vi "tilt.vi"(8 "error in (no error)":errorcluster, 10 "angle":dbl[unit], 11 "GenericTrajectory in":refnum<class "TrajectoryDL091126GenericVoxel.lvclass">) -> (0 "error out":errorcluster, 3 "GenericTrajectory out":refnum<class "TrajectoryDL091126GenericVoxel.lvclass">)   [LabVIEW 2010, in "TrajectoryDL091126GenericVoxel.lvclass"]
uses:
  TrajectoryDL091126GenericVoxel.lvclass
  TrajectoryDL091126GenericVoxel.lvclass/TrajectoryDL091126GenericVoxel.ctl
  common/legacy/axes.ctl
  common/enumerations/x_y_z_enumeration.ctl
  common/enumerations/functional_global_action_enum.ctl
  <vilib>/express/express arith-compare/Formula/XNode/ExpressFormulaBlockNode.xnode
  <vilib>/Analysis/Matrix/Numeric/Conversions/Array To Matrix - RA2.vi
  <vilib>/Analysis/baseanly.llb/Real A x B.vi
  <vilib>/Analysis/Matrix/Numeric/Conversions/Matrix To Array - RM.vi
  common/classes/ErrorController/ErrorController/class_data.vi
  <vilib>/Analysis/Matrix/NI_Matrix.lvlib
  <vilib>/Analysis/NI_AALBase.lvlib
  common/classes/ErrorController/ErrorController/ErrorController.lvclass
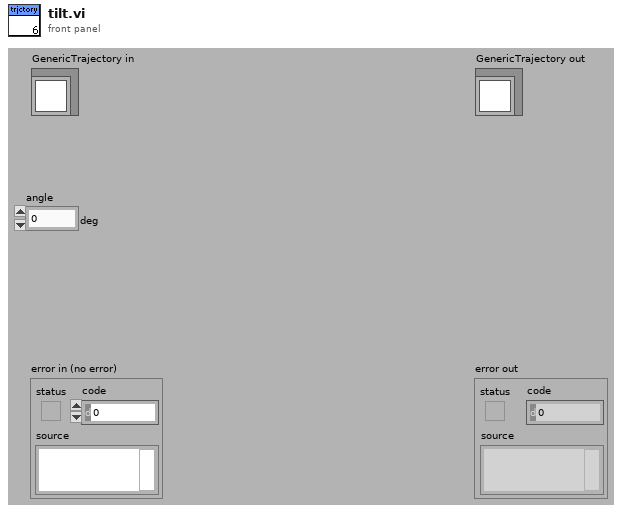
[diagram p1: front panel]
types:
  T1 = typedef "axes.ctl" = enum16{"x", "y", "z"}
  T2 = typedef "x_y_z_enumeration.ctl" = enum16{"x", "y", "z"}
  T3 = typedef "functional_global_action_enum.ctl" = enum16{"get", "set", "reset"}
  T4 = typedef "NI_Matrix.lvlib/RealMatrix.ctl" = dbl[][]
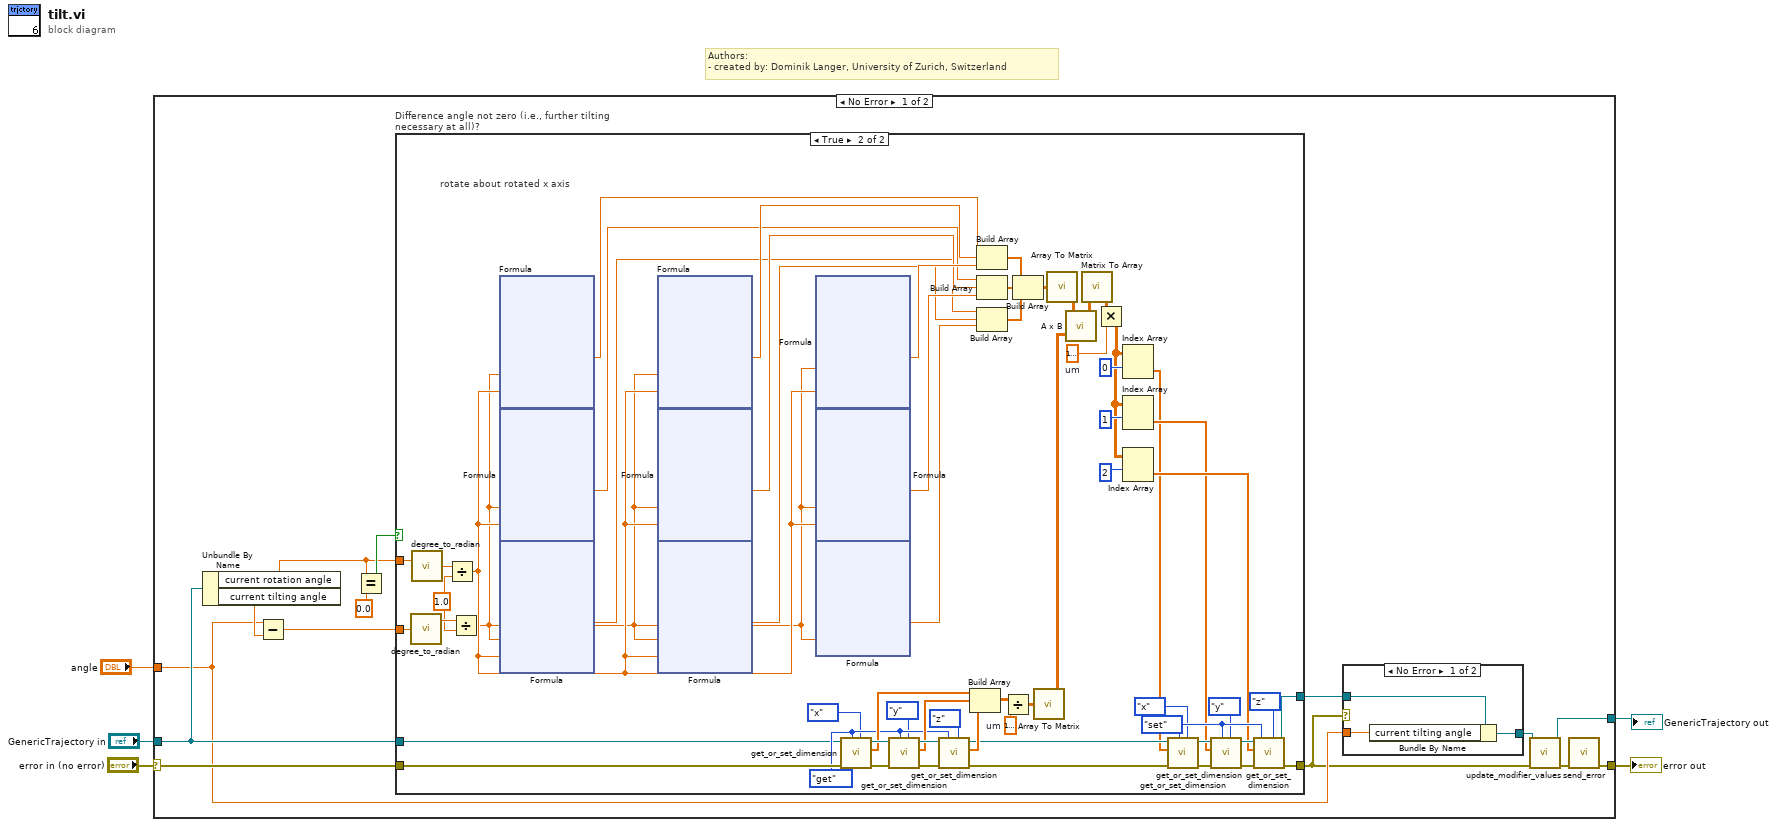
[diagram p0: block diagram]
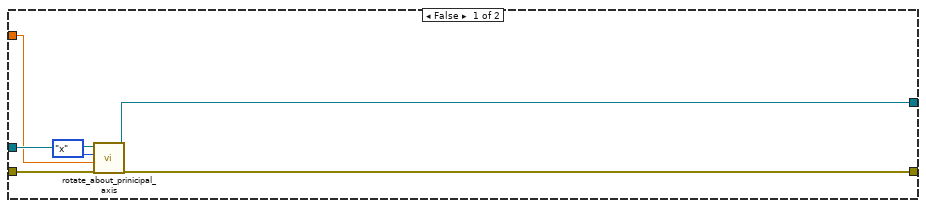
[diagram p3: hidden frame]
diagram:
  # "Authors: \n- created by: Dominik Langer, University of Zurich, Switzerland"
  n1 = case shown="No Error" "error in (no error)" {
    selector: "error in (no error)" -> [w15 w178]
    tunnel: [w6 w178] -> w4
    tunnel: [w8 w177] -> w2
    tunnel: "GenericTrajectory in" -> [w13 w177]
    tunnel: "angle" -> [w11 _]
    frame No Error {
      n2 = Unbundle By Name(w13) -> ("current rotation angle"=w14:dbl[unit], "current tilting angle"=w17:dbl[unit])
      n3 = Subtract(x=w11, y=w17) -> (x-y=w16:dbl[unit])
      n4 = Equal?(x=w14, y=dbl[unit] 0.0) -> (x = y?=w18:bool)
      n5 = case "Difference angle not zero (i.e., further tilting necessary at all)?" shown="True" w18 {
        tunnel: w16 -> [w24 w67]
        tunnel: w15 -> [w28 w60]
        tunnel: w13 -> [w26 w52]
        tunnel: w14 -> [_ w69]
        tunnel: [w25 w43] -> w12
        tunnel: [w27 w46] -> w10
        frame False {
          n6 = call-dynamic "rotate_about_prinicipal_axis.vi"("error in (no error)"=w28, "angle"=w24, "axis"=axes."x", "GenericTrajectory in"=w26) -> ("error out"=w27:errorcluster, "GenericTrajectory out"=w25:refnum<class "TrajectoryDL091126GenericVoxel.lvclass">)  [unwired: 6 out]
        }
        frame True {
          w49 = functional_global_action_enum."set" ("action")
          w54 = functional_global_action_enum."get" ("action")
          w66 = dbl[unit] 1.0 ("y")
          w38 = dbl[unit] 1e-06  # um
          w71 = dbl[unit] 1e-06  # um
          # "rotate about rotated x axis"
          n7 = call "degree_to_radian.vi"("angle in"=w67) -> ()  [unwired: 1 out]
          n8 = call "degree_to_radian.vi"("angle in"=w69) -> ("angle out"=w68:dbl[unit])
          n9 = Divide(x=w68, y=w66) -> (x/y=w70:dbl)
          n10 = Divide(x=w67, y=w66) -> (x/y=w65:dbl)
          n11 = xnode "Formula"("theta"=w65, "phi"=w70) -> ("Result"=w88:dbl)  [unwired: 1 in, 1 out]
          n12 = xnode "Formula"("theta"=w65, "phi"=w70) -> ("Result"=w84:dbl)  [unwired: 1 in, 1 out]
          n13 = xnode "Formula"("theta"=w65, "phi"=w70) -> ("Result"=w81:dbl)  [unwired: 1 in, 1 out]
          n14 = xnode "Formula"("theta"=w65, "phi"=w70) -> ("Result"=w86:dbl)  [unwired: 1 in, 1 out]
          n15 = xnode "Formula"("theta"=w65, "phi"=w70) -> ("Result"=w83:dbl)  [unwired: 1 in, 1 out]
          n16 = xnode "Formula"("theta"=w65, "phi"=w70) -> ("Result"=w80:dbl)  [unwired: 1 in, 1 out]
          n17 = xnode "Formula"("theta"=w65, "phi"=w70) -> ("Result"=w85:dbl)  [unwired: 1 in, 1 out]
          n18 = xnode "Formula"("theta"=w65, "phi"=w70) -> ("Result"=w82:dbl)  [unwired: 1 in, 1 out]
          n19 = xnode "Formula"("theta"=w65) -> ("Result"=w79:dbl)  [unwired: 1 in, 1 out]
          n20 = call-dynamic "get_or_set_dimension.vi"("dimension"=x_y_z_enumeration."x", "action"=w54, "error in (no error)"=w60, "GenericTrajectory in"=w52) -> ("error out"=w62:errorcluster, "pixel values out (single dimension)"=w59:dbl[unit][], "GenericTrajectory out"=w63:refnum<class "TrajectoryDL091126GenericVoxel.lvclass">)  [unwired: 2 in, 3 out]
          n21 = call-dynamic "get_or_set_dimension.vi"("dimension"=x_y_z_enumeration."y", "action"=w54, "error in (no error)"=w62, "GenericTrajectory in"=w63) -> ("error out"=w61:errorcluster, "pixel values out (single dimension)"=w58:dbl[unit][], "GenericTrajectory out"=w64:refnum<class "TrajectoryDL091126GenericVoxel.lvclass">)  [unwired: 2 in, 3 out]
          n22 = call-dynamic "get_or_set_dimension.vi"("dimension"=x_y_z_enumeration."z", "action"=w54, "error in (no error)"=w61, "GenericTrajectory in"=w64) -> ("error out"=w47:errorcluster, "pixel values out (single dimension)"=w57:dbl[unit][], "GenericTrajectory out"=w48:refnum<class "TrajectoryDL091126GenericVoxel.lvclass">)  [unwired: 2 in, 3 out]
          n23 = Build Array(w59, w58, w57) -> (w56:dbl[unit][][])
          n24 = Build Array(w88, w86, w85) -> (w87:dbl[])
          n25 = Build Array(w84, w83, w82) -> (w78:dbl[])
          n26 = Build Array(w81, w80, w79) -> (w77:dbl[])
          n27 = Divide(x=w56, y=w71) -> (x/y=w55:dbl[][])
          n28 = Build Array(w87, w78, w77) -> (w76:dbl[][])
          n29 = call-poly <vilib>:"Array To Matrix.vi"("Real 2D Array"=w55) -> ("Real Matrix"=w53:T4)
          n30 = call-poly <vilib>:"Array To Matrix.vi"("Real 2D Array"=w76) -> ("Real Matrix"=w75:T4)
          n31 = call-poly <vilib>:"A x B.vi"("B"=w53, "A"=w75) -> ("A x B"=w42:T4)  [unwired: 1 out]
          n32 = call-poly <vilib>:"Matrix To Array.vi"("Real Matrix"=w42) -> ("Real 2D Array"=w39:dbl[][])
          n33 = Multiply(x=w39, y=w38) -> (x*y=w40:dbl[unit][][])
          n34 = Index Array(array=w40, index (row)=0) -> (element=w36:dbl[unit][])  [unwired: 1 in]
          n35 = Index Array(array=w40, index (row)=1) -> (element=w37:dbl[unit][])  [unwired: 1 in]
          n36 = Index Array(array=w40, index (row)=2) -> (element=w41:dbl[unit][])  [unwired: 1 in]
          n37 = call-dynamic "get_or_set_dimension.vi"("dimension"=x_y_z_enumeration."x", "action"=w49, "error in (no error)"=w47, "pixel values in (single dimension)"=w36, "GenericTrajectory in"=w48) -> ("error out"=w45:errorcluster, "GenericTrajectory out"=w51:refnum<class "TrajectoryDL091126GenericVoxel.lvclass">)  [unwired: 1 in, 4 out]
          n38 = call-dynamic "get_or_set_dimension.vi"("dimension"=x_y_z_enumeration."y", "action"=w49, "error in (no error)"=w45, "pixel values in (single dimension)"=w37, "GenericTrajectory in"=w51) -> ("error out"=w44:errorcluster, "GenericTrajectory out"=w50:refnum<class "TrajectoryDL091126GenericVoxel.lvclass">)  [unwired: 1 in, 4 out]
          n39 = call-dynamic "get_or_set_dimension.vi"("dimension"=x_y_z_enumeration."z", "action"=w49, "error in (no error)"=w44, "pixel values in (single dimension)"=w41, "GenericTrajectory in"=w50) -> ("error out"=w46:errorcluster, "GenericTrajectory out"=w43:refnum<class "TrajectoryDL091126GenericVoxel.lvclass">)  [unwired: 1 in, 4 out]
        }
      }
      n40 = case shown="No Error" w10 {
        tunnel: w12 -> [w22 w23]
        tunnel: [w21 w23] -> w9
        tunnel: w11 -> [w20 _]
        frame No Error {
          n41 = Bundle By Name(cluster=w22, "current tilting angle"=w20) -> (w21:refnum<class "TrajectoryDL091126GenericVoxel.lvclass">)
        }
        frame Error {
        }
      }
      n42 = call-dynamic "update_modifier_values.vi"("TrajectoryDL091126GenericVoxel in"=w9, "error in (no error)"=w10) -> ("TrajectoryDL091126GenericVoxel out"=w8:refnum<class "TrajectoryDL091126GenericVoxel.lvclass">, "error out"=w7:errorcluster)  [unwired: 9 in, 3 out]
      n43 = call "send_error.vi"("error in (no error)"=w7) -> ("error out"=w6:errorcluster)  [unwired: 10 in]
    }
    frame Error {
    }
  }
  "error out" <- w4
  "GenericTrajectory out" <- w2
